vi "Add Available Worker.vi"(8 "error in":errorcluster, 10 "Worker":refnum<class "Message Enqueuer.lvclass">, 11 "Work Dispatcher in":refnum<class "Work Dispatcher.lvclass">) -> (0 "error out":errorcluster, 3 "Work Dispatcher out":refnum<class "Work Dispatcher.lvclass">)   [LabVIEW 2023, in "Work Dispatcher.lvlib" / "Work Dispatcher.lvclass"]
doc: "Add a worker to the available workers queue."
uses:
  Work Dispatcher.lvclass
  c:/dev/_r/4/eng/lv-core/lvpostprocessingd/lv_mc_x86_64/dist_i386/vi.lib/ActorFramework/Actor/Actor.lvclass
  <vilib>/ActorFramework/Message Enqueuer/Message Enqueuer.lvclass
  <vilib>/ActorFramework/Actor/Actor.lvclass/Actor.ctl
  <vilib>/ActorFramework/Message Enqueuer/Message Enqueuer.lvclass/Message Enqueuer.ctl
  Work Dispatcher.lvclass/Work Dispatcher.ctl
  Person Messages/Process Job Msg/Process Job Msg.lvclass/Process Job Msg.ctl
  Work Dispatcher Messages/Add Task Msg/Add Task Msg.lvclass/Add Task Msg.ctl
  <vilib>/ActorFramework/Message Enqueuer/Init from Existing Queue.vi
  <vilib>/ActorFramework/Message Enqueuer/Enqueue.vi
  Person Messages/Process Job Msg/Process Job Msg.lvclass
  c:/dev/_r/4/eng/lv-core/lvpostprocessingd/lv_mc_x86_64/dist_i386/vi.lib/ActorFramework/Message/Message.lvclass
  Work Dispatcher Messages/Add Task Msg/Add Task Msg.lvclass
  <vilib>/ActorFramework/Message Priority Queue/Priority Enqueue.vi
  <vilib>/ActorFramework/Actor/Actor.lvclass
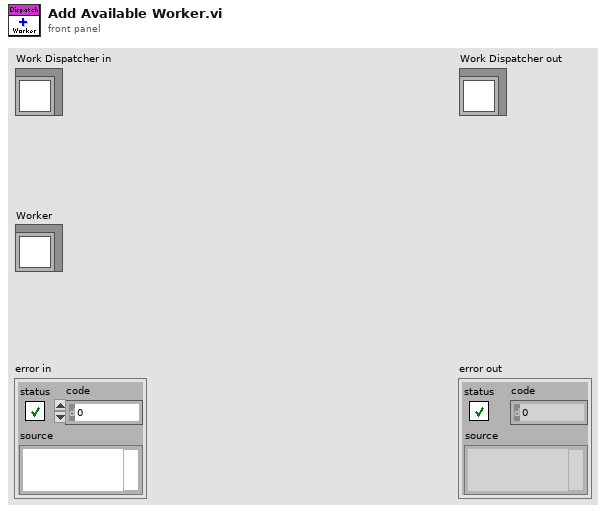
[diagram p1: front panel]
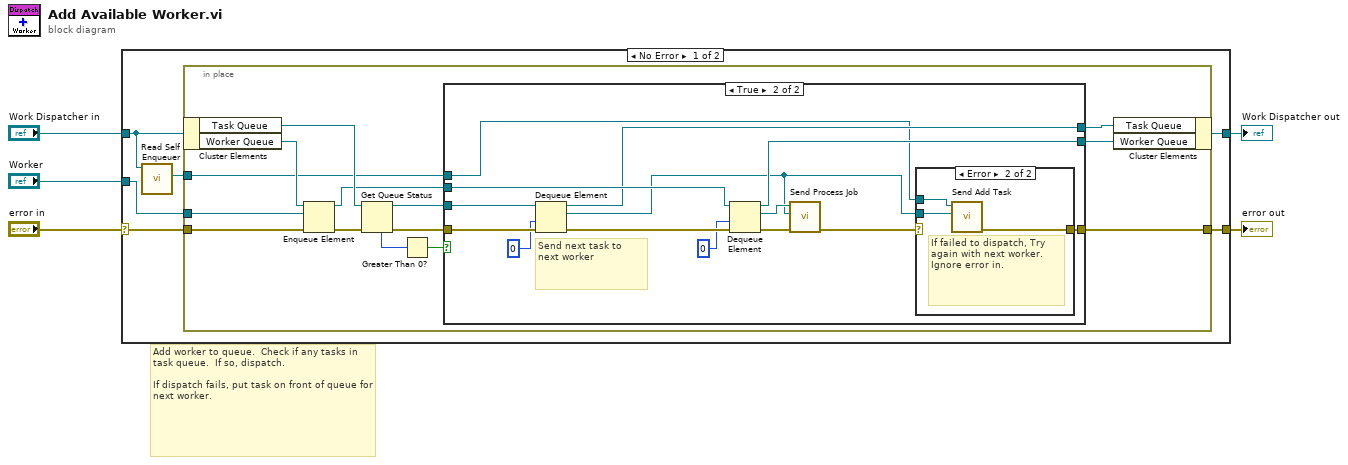
[diagram p0: block diagram]
diagram:
  # "Add worker to queue.  Check if any tasks in task queue.  If so, dispatch.\n\nIf dispatch fails, put task on front of queue for next worker."
  n1 = case shown="No Error" "error in" {
    selector: "error in" -> [w10 w48]
    tunnel: [w9 w48] -> w4
    tunnel: [w8 w47] -> w2
    tunnel: "Work Dispatcher in" -> [w7 w47]
    tunnel: "Worker" -> [w11 _]
    frame No Error {
      n2 = call <vilib>:"Read Self Enqueuer.vi"("Actor"=w7) -> ("Self Enqueuer"=w6:refnum<class "Message Enqueuer.lvclass">)  [unwired: 10 in]
      n3 = in-place "In Place Element Structure" {
        in-place-border: w11 -> [w24]
        in-place-border: w10 -> [w23]
        in-place-border: [w15] -> w9
        in-place-border: w6 -> [w12]
        n4 = in-place-cluster #1 ("Unbundle / Bundle Elements")(w7) -> ("Task Queue"=w22:refnum<queue>, "Worker Queue"=w25:refnum<queue>)
        n5 = Enqueue Element(queue=w25, element=w24, error in (no error)=w23) -> (queue out=w18:refnum<queue>, error out=w16:errorcluster)  [unwired: 1 in, 1 out]
        n6 = Get Queue Status(queue=w22, error in (no error)=w16) -> (queue out=w19:refnum<queue>, error out=w17:errorcluster, # elements in queue=w21:i32)  [unwired: 1 in, 5 out]
        n7 = Greater Than 0?(x=w21) -> (x > 0?=w20:bool)
        n8 = case shown="True" w20 {
          tunnel: w19 -> [w28 w42]
          tunnel: w18 -> [w26 w41]
          tunnel: w17 -> [w27 w39]
          tunnel: [w27 w31] -> w15
          tunnel: [w26 w38] -> w14
          tunnel: [w28 w30] -> w13
          tunnel: w12 -> [_ w29]
          frame False {
          }
          frame True {
            # "Send next task to next worker"
            n9 = Dequeue Element(queue=w42, timeout in ms (-1)=0, error in (no error)=w39) -> (queue out=w30:refnum<queue>, element=w32:refnum<class>, error out=w40:errorcluster)  [unwired: 1 out]
            n10 = Dequeue Element(queue=w41, timeout in ms (-1)=0, error in (no error)=w40) -> (queue out=w38:refnum<queue>, element=w36:refnum<class "Message Enqueuer.lvclass">, error out=w37:errorcluster)  [unwired: 1 out]
            n11 = call "Send Process Job.vi"("error in (no error)"=w37, "Task"=w32, "Message Enqueuer"=w36) -> ("error out"=w33:errorcluster)  [unwired: 7 in, 1 out]
            n12 = case shown="Error" w33 {
              selector: w33 -> [w43 _]
              tunnel: w32 -> [_ w45]
              tunnel: [w43 w46] -> w31
              tunnel: w29 -> [_ w44]
              frame No Error {
              }
              frame Error {
                # "If failed to dispatch, Try again with next worker.  Ignore error in."
                n13 = call "Send Add Task.vi"("Task"=w45, "Message Enqueuer"=w44) -> ("error out"=w46:errorcluster)  [unwired: 8 in, 1 out]
              }
            }
          }
        }
        n14 = in-place-cluster #1 ("Unbundle / Bundle Elements")("Task Queue"=w13, "Worker Queue"=w14) -> (w8:refnum<class "Work Dispatcher.lvclass">)
      }
    }
    frame Error {
    }
  }
  "error out" <- w4
  "Work Dispatcher out" <- w2
